vi "ScanPanelTHz.vi"(8 "error in (no error)":errorcluster caption="entrée d'erreur (pas d'erreur)", 11 "KlingerMotor.lvclass":refnum<class "KlingerMotor.lvclass">) -> (0 "error out":errorcluster caption="sortie d'erreur", 3 "KlingerMotor.lvclass Out":refnum<class "KlingerMotor.lvclass">)   [LabVIEW 2019, in "KlingerMotor.lvclass"]
uses:
  KlingerMotor.lvclass
  C:/Programmes Labview/LabScanV1A/DevicesClass/BaseDevice/BaseDevice.lvclass
  KlingerMotor.lvclass/KlingerMotor.ctl
  BaseDevice/ScanPos.ctl
  <userlib>/KlingerV2/KlingerV2 ConvUnitSgl.vi
panel:
  in  "UpdateScanTime":bool
  in  "MainProgQ":refnum<queue>
  in  "MainProgQEvent":refnum<user-event>
  out "Debut (ps)":dbl caption="Début (ps)"
  out "Fin (ps)":dbl caption="Fin"
  out "Increment (ps)":dbl=1.0 caption="Increment" min=1e-06 step=1e-06
  in  "Reinit":bool caption="Reinitializer à la fin"
  in  "Bidirectionel":bool
  out "Positions":dbl[](array[numeric])
  in  "Modèle":u16(ring) caption="Modèle de Balayage"
  in  "CréerMod":bool
  in  "Debut":dbl caption="Début(mm)"
  in  "Fin":dbl
  in  "Increment":dbl=1.0 min=1e-06 step=1e-06
  in  "ModRap":bool caption="Modèle Rapide"
  in  "Stop":bool
  out "Init Program":bool
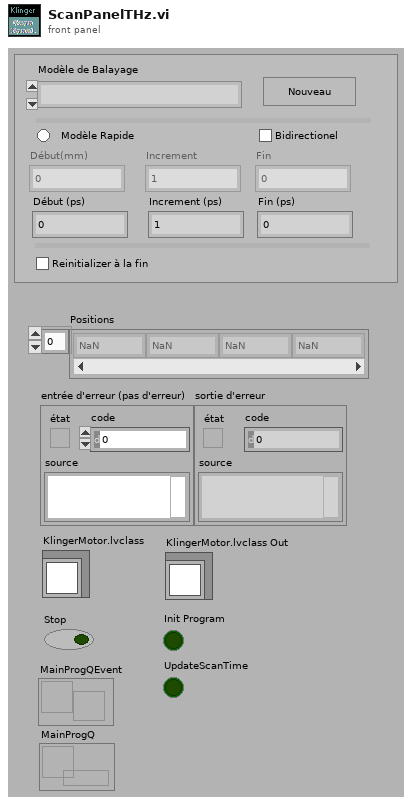
[diagram p1: front panel]
types:
  T1 = enum16{"Enable", "Disable", "DisAndGrayed", "ReinitToDefVal"}
  T2 = typedef "ScanPos.ctl" = cluster{"Debut":dbl, "Increment":dbl, "Fin":dbl, "Positions":dbl[], "Bidir":bool, "ModelRap":bool}
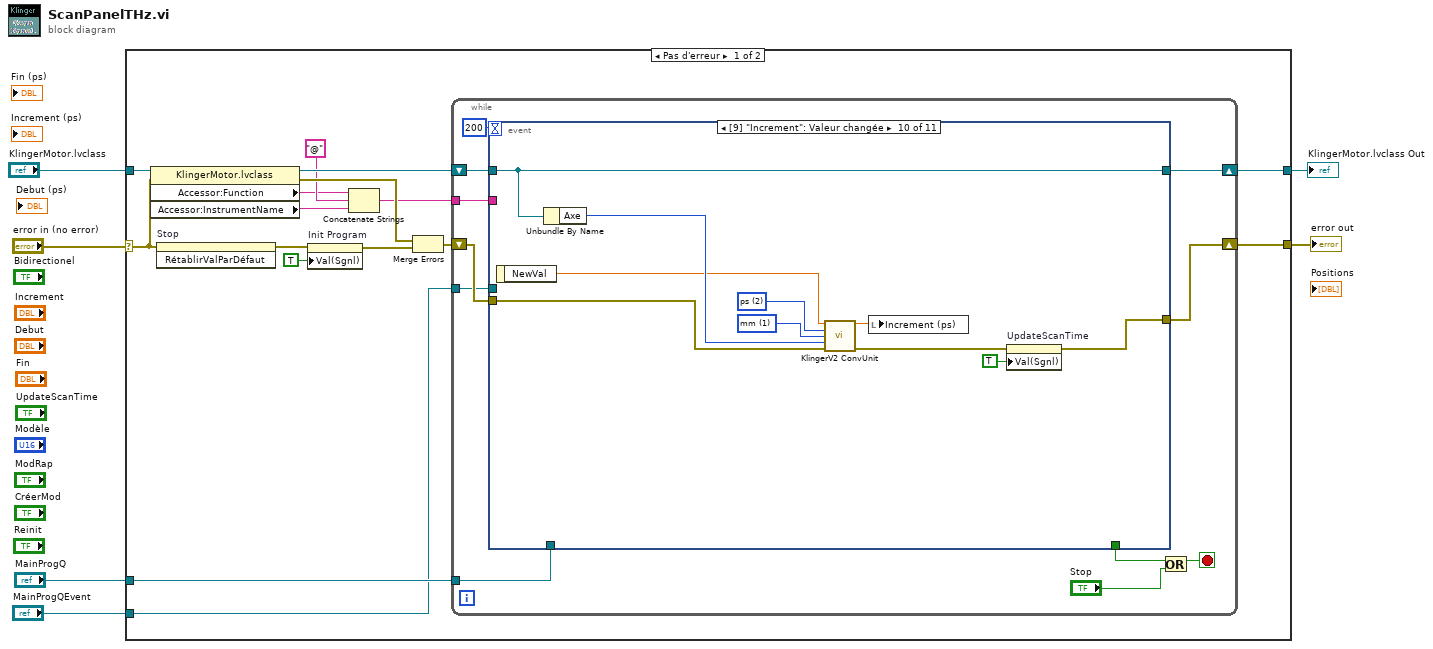
[diagram p0: block diagram]
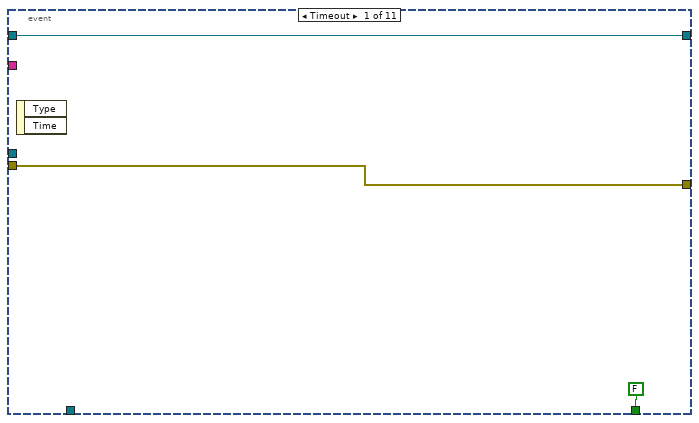
[diagram p2: hidden frame]
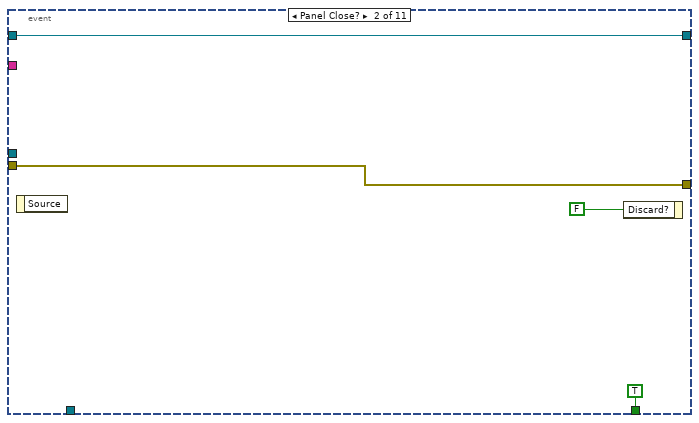
[diagram p3: hidden frame]
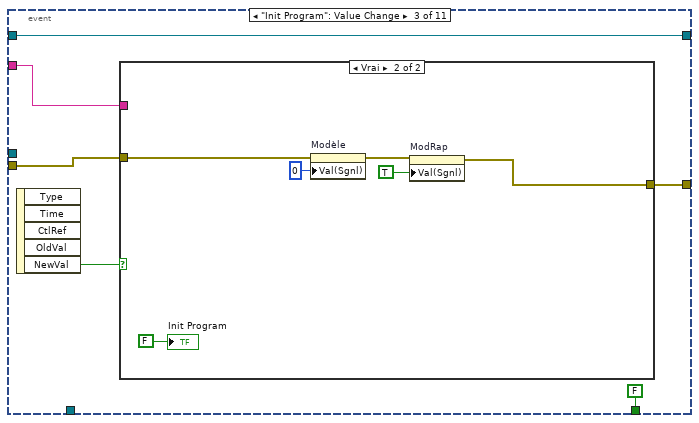
[diagram p4: hidden frame]
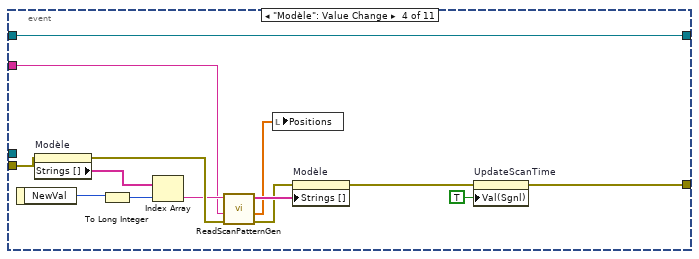
[diagram p6: hidden frame]
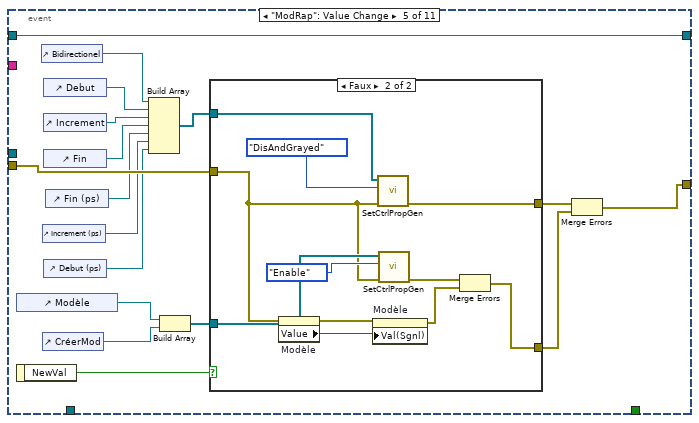
[diagram p7: hidden frame]
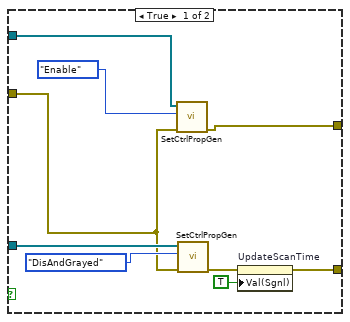
[diagram p8: hidden frame]
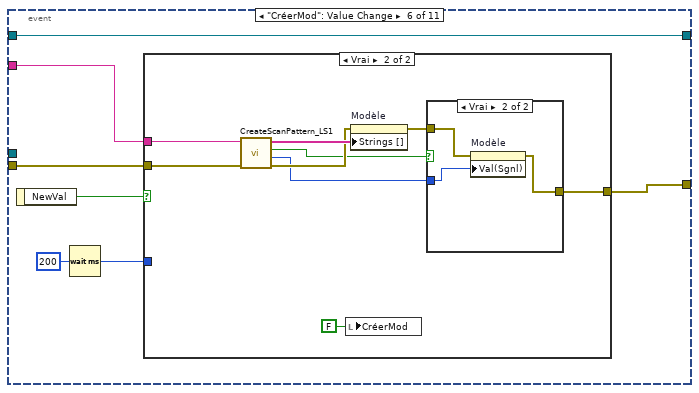
[diagram p9: hidden frame]
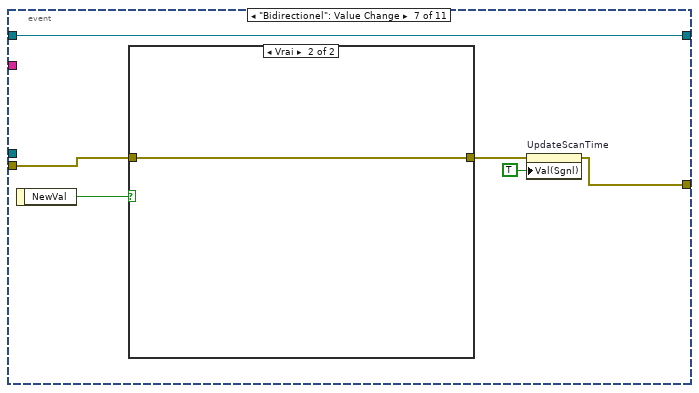
[diagram p12: hidden frame]
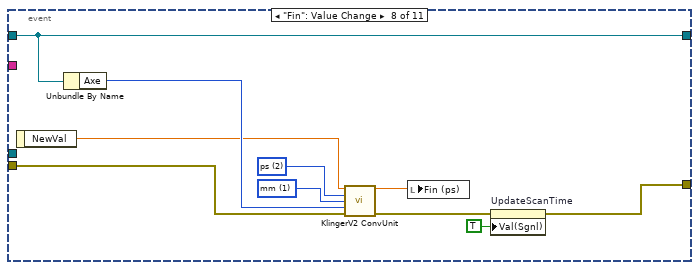
[diagram p14: hidden frame]
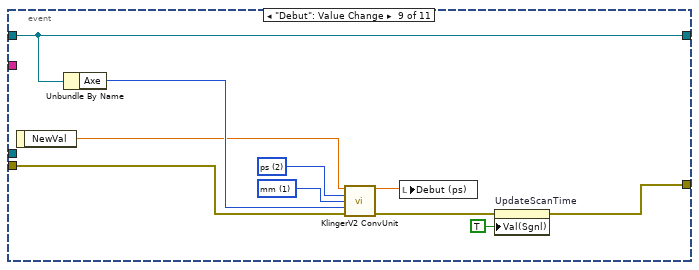
[diagram p15: hidden frame]
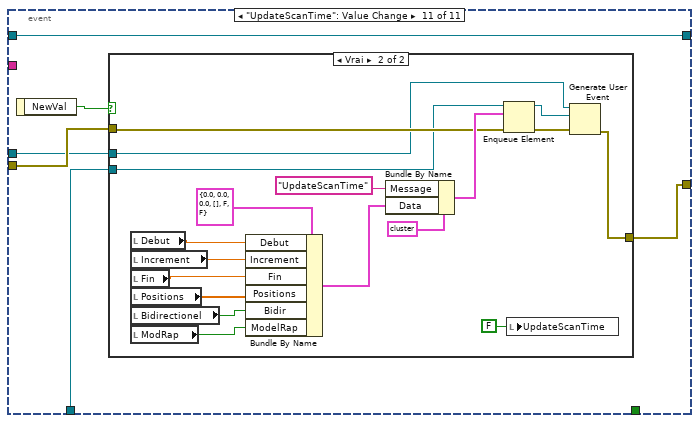
[diagram p16: hidden frame]
diagram:
  n1 = case shown="Pas d'erreur" "error in (no error)" {
    selector: "error in (no error)" -> [w16 w190]
    tunnel: [w22 w190] -> w5
    tunnel: "KlingerMotor.lvclass" -> [w21 w189]
    tunnel: [w19 w189] -> w3
    tunnel: "MainProgQ" -> [w8 _]
    tunnel: "MainProgQEvent" -> [w7 _]
    frame No Error {
      n2 = property class="KlingerMotor.lvclass"(reference=w21, error in=w16) -> (reference out=w17:refnum<class "KlingerMotor.lvclass">, error out=w14:errorcluster, "Accessor:Function"=w11:string, "Accessor:InstrumentName"=w10:string)
      n3 = invoke on="Stop" class="Bool (strict)" method="RétablirValParDéfaut"(error in=w16) -> (error out=w18:errorcluster)  [unwired: 2 in, 2 out]
      n4 = property on="Init Program" class="Bool (strict)"(error in=w18, "Val(Sgnl)"=TRUE ("Valeur (Signalisation)")) -> (error out=w15:errorcluster)  [unwired: 1 in, 1 out]
      n5 = Concatenate Strings(w11, "@" ("chaîne"), w10) -> (w9:string)
      n6 = Merge Errors(w14, w15) -> (w13:errorcluster)
      n7 = while {
        shift-right: [w32] -> w22
        shift-left: w13 -> [w25]
        shift-right: [w29] -> w19
        shift-left: w17 -> [w31]
        tunnel: w9 -> [w26]
        tunnel: w8 -> [w24]
        tunnel: w7 -> [w23]
        stop <- w28 stop-if-true
        n8 = event shown="[9] \"Increment\": Valeur changée" {
          selector: _ -> [_ _ _ _ _ _ _ _ _ _ _]
          dyn-events: _ -> [_ _ _ _ _ _ _ _ _ _ _]
          timeout: 200 -> [_ _ _ _ _ _ _ _ _ _ _]
          tunnel: w25 -> [w34 w38 w45 w67 w78 w106 w130 w139 w149 w159 w167]
          tunnel: [w34 w38 w44 w55 w72 w105 w127 w135 w145 w155 w168] -> w32
          tunnel: w31 -> [w35 w37 w43 w58 w77 w108 w129 w143 w153 w163 w166]
          tunnel: [FALSE TRUE FALSE _ _ _ _ _ _ _ _] -> w30
          tunnel: [w35 w37 w43 w58 w77 w108 w129 w143 w153 w163 w166] -> w29
          tunnel: w26 -> [_ _ w41 w57 _ w107 _ _ _ _ _]
          tunnel: w24 -> [_ _ _ _ _ _ _ _ _ _ w165]
          tunnel: w23 -> [_ _ _ _ _ _ _ _ _ _ w164]
          event Timeout {
            n9 = event-data() -> ()  [unwired: 1 in, 2 out]
          }
          event Panel Close? {
            n10 = event-data() -> ()  [unwired: 1 in, 1 out]
            n11 = event-data("Discard?"=FALSE ("Rejeter ?")) -> ()  [unwired: 1 in, 1 out]
          }
          event "Init Program": Value Change {
            n12 = event-data() -> ("NewVal"=w46:bool)  [unwired: 1 in, 4 out]
            n13 = case shown="Vrai" w46 {
              tunnel: w41 -> [_ _]
              tunnel: w45 -> [w47 w50]
              tunnel: [w47 w52] -> w44
              frame False {
              }
              frame True {
                n14 = property on="Modèle" class="MDér (strict)"(error in=w50, "Val(Sgnl)"=u16 0 ("Valeur (Signalisation)")) -> (error out=w49:errorcluster)  [unwired: 1 in, 1 out]
                n15 = property on="ModRap" class="Bool (strict)"(error in=w49, "Val(Sgnl)"=TRUE ("ModRap")) -> (error out=w52:errorcluster)  [unwired: 1 in, 1 out]
                "Init Program" <- FALSE
              }
            }
          }
          event "Modèle": Value Change {
            n16 = event-data() -> ("NewVal"=w65:u16)  [unwired: 1 in]
            n17 = property on="Modèle" class="MDér (strict)"(error in=w67) -> (error out=w63:errorcluster, "Strings []"=w64:string[])  [unwired: 1 in, 1 out]
            n18 = To Long Integer(number=w65) -> (32bit integer=w66:i32)
            n19 = Index Array(array=w64, index=w66) -> (element=w62:string)
            n20 = call <userlib>:"ReadScanPatternGen.vi"("Error in"=w63, "VarParam"=w57, "Modèle"=w62) -> ("Error out"=w60:errorcluster, "Positions"=w59:dbl[], "Modèles"=w61:string[])  [unwired: 2 in]
            n21 = local write "Positions"(w59) -> ()
            n22 = property on="Modèle" class="MDér (strict)"(error in=w60, "Strings []"=w61) -> (error out=w56:errorcluster)  [unwired: 1 in, 1 out]
            n23 = property on="UpdateScanTime" class="Bool (strict)"(error in=w56, "Val(Sgnl)"=TRUE ("Value (Signaling)")) -> (error out=w55:errorcluster)  [unwired: 1 in, 1 out]
          }
          event "ModRap": Value Change {
            n24 = control-ref of="Modèle"() -> (w80:refnum<vi>)
            n25 = event-data() -> ("NewVal"=w76:bool)  [unwired: 1 in]
            n26 = control-ref of="Bidirectionel"() -> (w71:refnum<vi>)
            n27 = control-ref of="Increment (ps)"() -> (w69:refnum<vi>)
            n28 = control-ref of="CréerMod"() -> (w79:refnum<vi>)
            n29 = control-ref of="Debut"() -> (w84:refnum<vi>)
            n30 = control-ref of="Increment"() -> (w83:refnum<vi>)
            n31 = control-ref of="Fin"() -> (w82:refnum<vi>)
            n32 = control-ref of="Debut (ps)"() -> (w68:refnum<vi>)
            n33 = control-ref of="Fin (ps)"() -> (w70:refnum<vi>)
            n34 = Build Array(w71, w84, w83, w82, w70, w69, w68) -> (w81:refnum<vi>[])
            n35 = Build Array(w80, w79) -> (w75:refnum<vi>[])
            n36 = case shown="Faux" w76 {
              tunnel: w81 -> [w93 w104]
              tunnel: w78 -> [w89 w98]
              tunnel: w75 -> [w90 w101]
              tunnel: [w88 w100] -> w74
              tunnel: [w86 w94] -> w73
              frame True {
                n37 = call <userlib>:"SetCtrlPropGen.vi"("Error in"=w89, "Énum"=T1."Enable", "Controls"=w93) -> ("Error out"=w88:errorcluster)  [unwired: 3 in, 1 out]
                n38 = call <userlib>:"SetCtrlPropGen.vi"("Error in"=w89, "Énum"=T1."DisAndGrayed", "Controls"=w90) -> ("Error out"=w87:errorcluster)  [unwired: 3 in, 1 out]
                n39 = property on="UpdateScanTime" class="Bool (strict)"(error in=w87, "Val(Sgnl)"=TRUE ("Value (Signaling)")) -> (error out=w86:errorcluster)  [unwired: 1 in, 1 out]
              }
              frame False {
                n40 = property on="Modèle" class="MDér (strict)"(error in=w98) -> (error out=w97:errorcluster, "Value"=w99:u16)  [unwired: 1 in, 1 out]
                n41 = property on="Modèle" class="MDér (strict)"(error in=w97, "Val(Sgnl)"=w99) -> (error out=w95:errorcluster)  [unwired: 1 in, 1 out]
                n42 = call <userlib>:"SetCtrlPropGen.vi"("Error in"=w98, "Énum"=T1."DisAndGrayed", "Controls"=w104) -> ("Error out"=w100:errorcluster)  [unwired: 3 in, 1 out]
                n43 = call <userlib>:"SetCtrlPropGen.vi"("Error in"=w98, "Énum"=T1."Enable", "Controls"=w101) -> ("Error out"=w96:errorcluster)  [unwired: 3 in, 1 out]
                n44 = Merge Errors(w96, w95) -> (w94:errorcluster)
              }
            }
            n45 = Merge Errors(w74, w73) -> (w72:errorcluster)
          }
          event "CréerMod": Value Change {
            n46 = event-data() -> ("NewVal"=w111:bool)  [unwired: 1 in]
            n47 = Wait (ms)(milliseconds to wait=u32 200 ("attente (ms)")) -> (millisecond timer value=w110:u32)
            n48 = case shown="Vrai" w111 {
              tunnel: w110 -> [_ _]
              tunnel: w107 -> [_ w120]
              tunnel: w106 -> [w112 w119]
              tunnel: [w112 w115] -> w105
              frame False {
              }
              frame True {
                n49 = call "CreateScanPattern_LS1.vi"("Error in"=w119, "VarParam"=w120) -> ("Error out"=w117:errorcluster, "ModèleSauv"=w113:i32, "SavedOK"=w114:bool, "Modèles out"=w118:string[])  [unwired: 6 in]
                n50 = local write "CréerMod"(FALSE ("CréerMod")) -> ()
                n51 = property on="Modèle" class="MDér (strict)"(error in=w117, "Strings []"=w118) -> (error out=w116:errorcluster)  [unwired: 1 in, 1 out]
                n52 = case shown="Vrai" w114 {
                  tunnel: w116 -> [w122 w125]
                  tunnel: [w122 w124] -> w115
                  tunnel: w113 -> [_ w123]
                  frame False {
                  }
                  frame True {
                    n53 = property on="Modèle" class="MDér (strict)"(error in=w125, "Val(Sgnl)"=w123) -> (error out=w124:errorcluster)  [unwired: 1 in, 1 out]
                  }
                }
              }
            }
          }
          event "Bidirectionel": Value Change {
            n54 = event-data() -> ("NewVal"=w131:bool)  [unwired: 1 in]
            n55 = case shown="Vrai" w131 {
              tunnel: [w132 w133] -> w128
              tunnel: w130 -> [w132 w133]
              frame False {
              }
              frame True {
              }
            }
            n56 = property on="UpdateScanTime" class="Bool (strict)"(error in=w128, "Val(Sgnl)"=TRUE ("Value (Signaling)")) -> (error out=w127:errorcluster)  [unwired: 1 in, 1 out]
          }
          event "Fin": Value Change {
            w140 = u8 2 items=["Pas", "mm", "ps", "Degré (°)"] ("UnitDem")
            w141 = u8 1 items=["Pas", "mm", "ps", "Degré (°)"] ("UnitAct")
            n57 = event-data() -> ("NewVal"=w138:dbl)  [unwired: 1 in]
            n58 = Unbundle By Name(w143) -> ("Axe"=w142:u8)
            n59 = call-poly <userlib>:"KlingerV2 ConvUnit.vi"("ParamAct"=w138, "UnitDem"=w140, "UnitAct"=w141, "Axe"=w142, "error in"=w139) -> ("ParamDem"=w137:dbl, "error out"=w136:errorcluster)  [unwired: 9 in]
            n60 = local write "Fin (ps)"(w137) -> ()
            n61 = property on="UpdateScanTime" class="Bool (strict)"(error in=w136, "Val(Sgnl)"=TRUE ("Value (Signaling)")) -> (error out=w135:errorcluster)  [unwired: 1 in, 1 out]
          }
          event "Debut": Value Change {
            w150 = u8 2 items=["Pas", "mm", "ps", "Degré (°)"] ("UnitDem")
            w151 = u8 1 items=["Pas", "mm", "ps", "Degré (°)"] ("UnitAct")
            n62 = event-data() -> ("NewVal"=w148:dbl)  [unwired: 1 in]
            n63 = Unbundle By Name(w153) -> ("Axe"=w152:u8)
            n64 = call-poly <userlib>:"KlingerV2 ConvUnit.vi"("ParamAct"=w148, "UnitDem"=w150, "UnitAct"=w151, "Axe"=w152, "error in"=w149) -> ("ParamDem"=w147:dbl, "error out"=w146:errorcluster)  [unwired: 9 in]
            n65 = local write "Debut (ps)"(w147) -> ()
            n66 = property on="UpdateScanTime" class="Bool (strict)"(error in=w146, "Val(Sgnl)"=TRUE ("Value (Signaling)")) -> (error out=w145:errorcluster)  [unwired: 1 in, 1 out]
          }
          event "Increment": Value Change {
            w160 = u8 2 items=["Pas", "mm", "ps", "Degré (°)"] ("UnitDem")
            w161 = u8 1 items=["Pas", "mm", "ps", "Degré (°)"] ("UnitAct")
            n67 = event-data() -> ("NewVal"=w158:dbl)  [unwired: 1 in]
            n68 = Unbundle By Name(w163) -> ("Axe"=w162:u8)
            n69 = call-poly <userlib>:"KlingerV2 ConvUnit.vi"("ParamAct"=w158, "UnitDem"=w160, "UnitAct"=w161, "Axe"=w162, "error in"=w159) -> ("ParamDem"=w157:dbl, "error out"=w156:errorcluster)  [unwired: 9 in]
            n70 = local write "Increment (ps)"(w157) -> ()
            n71 = property on="UpdateScanTime" class="Bool (strict)"(error in=w156, "Val(Sgnl)"=TRUE ("Value (Signaling)")) -> (error out=w155:errorcluster)  [unwired: 1 in, 1 out]
          }
          event "UpdateScanTime": Value Change {
            n72 = event-data() -> ("NewVal"=w169:bool)  [unwired: 1 in]
            n73 = case shown="Vrai" w169 {
              tunnel: [w170 w179] -> w168
              tunnel: w167 -> [w170 w180]
              tunnel: w165 -> [_ w178]
              tunnel: w164 -> [_ w177]
              frame False {
              }
              frame True {
                n74 = local read "Debut"() -> (w174:dbl)
                n75 = local read "Increment"() -> (w175:dbl)
                n76 = local read "Fin"() -> (w176:dbl)
                n77 = local read "Positions"() -> (w173:dbl[])
                n78 = local read "Bidirectionel"() -> (w172:bool)
                n79 = local read "ModRap"() -> (w171:bool)
                n80 = Bundle By Name(cluster=T2 {"Debut"=0.0, "Increment"=0.0, "Fin"=0.0, "Positions"=[], "Bidir"=FALSE, "ModelRap"=FALSE}, "Debut"=w174, "Increment"=w175, "Fin"=w176, "Positions"=w173, "Bidir"=w172, "ModelRap"=w171) -> (w187:T2)
                n81 = Bundle By Name(cluster=cluster{"Message":string, "Data":variant, i32} {"Message"="", "Data"=variant, 0} ("élément"), "Message"="UpdateScanTime", "Data"=w187) -> (w182:cluster{"Message":string, "Data":variant, i32})
                n82 = Enqueue Element(queue=w178, element=w182, error in (no error)=w180) -> (queue out=w183:refnum<queue>, error out=w184:errorcluster)  [unwired: 1 in, 1 out]
                n83 = local write "UpdateScanTime"(FALSE ("UpdateScanTime")) -> ()
                n84 = Generate User Event(user event=w177, event data cluster=w183, error in=w184) -> (error out=w179:errorcluster)  [unwired: 1 in, 1 out]
              }
            }
          }
        }
        n85 = Or(x=w30, y="Stop") -> (x .or. y?=w28:bool)
      }
    }
    frame Error {
    }
  }
  "error out" <- w5
  "KlingerMotor.lvclass Out" <- w3
